vi "io.debouncer.vi"(0 "input":bool) -> (2 "output":bool)   [LabVIEW 2019]
panel:
  in  "debouncer (ms)":u16=10
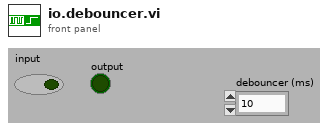
[diagram p1: front panel]
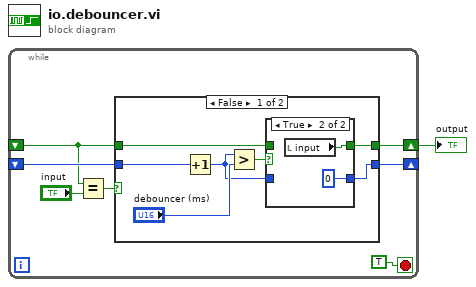
[diagram p0: block diagram]
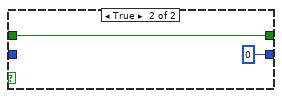
[diagram p3: hidden frame]
diagram:
  n1 = while {
    shift-right: [w4] -> w1
    shift-left: _ -> [w2]
    shift-right: [w6] -> _
    shift-left: _ -> [w7]
    stop <- TRUE stop-if-true
    n2 = Equal?(x=w2, y="input") -> (x = y?=w5:bool)
    n3 = case shown="False" w5 {
      tunnel: w7 -> [w15 _]
      tunnel: [w11 u16 0] -> w6
      tunnel: [w12 w20] -> w4
      tunnel: w2 -> [w9 w20]
      frame False {
        n4 = Increment(x=w15) -> (x+1=w10:u16)
        n5 = Greater?(x=w10, y="debouncer (ms)") -> (0:w13:bool)
        n6 = case shown="True" w13 {
          tunnel: [w16 w19] -> w12
          tunnel: [w17 u16 0] -> w11
          tunnel: w10 -> [w17 _]
          tunnel: w9 -> [w16 _]
          frame False {
          }
          frame True {
            n7 = local read "input"() -> (w19:bool)
          }
        }
      }
      frame True {
      }
    }
  }
  "output" <- w1
